vi "Teleop.vi"(10 "Match Info":T1={"Autonomous Elapsed Seconds"=0.0, "TeleOp Elapsed Seconds"=0.0, "Disabled Elapsed Seconds"=0.0, "Visited Autonomous"=FALSE, "Visited TeleOp"=FALSE, "Visited Disabled"=FALSE, "Autonomous Settings"={"Autonomous Style"=enum."Independent", "VI Refnum"=refnum}}, 11 "Call Context":T2) -> ()   [LabVIEW 2015]
doc: "This VI is called for each enabled TeleOp packet received from the DS. It is typically used to read from joysticks and other inputs and update I/O or setpoints for timed control loops. It should complete and return within 20 milliseconds or risk missing DS packets."
uses:
  <vilib>/Rock Robotics/WPI/DriverStation/WPI_DriverStationDerivedRobotMode.ctl
  <vilib>/Rock Robotics/WPI/DriverStation/WPI_DriverStationMatch Info.ctl
  <vilib>/Rock Robotics/WPI/Solenoid/WPI_SolenoidValue.ctl
  <vilib>/Rock Robotics/WPI/Utilities/WPI_GetSetVariantRefNum.vi
  <vilib>/Rock Robotics/Network Tables/NT Write Boolean Array.vi
  <vilib>/Rock Robotics/Network Tables/NT Write Numeric Array.vi
  <vilib>/Rock Robotics/WPI/RobotDrive/WPI_RobotDriveArcadeDrive_Standard(NoSaturation).vi
  <vilib>/Rock Robotics/WPI/Solenoid/Deprecated/WPI_SolenoidGetBool.vi
  <vilib>/Rock Robotics/WPI/Solenoid/WPI_SolenoidSetEnum.vi
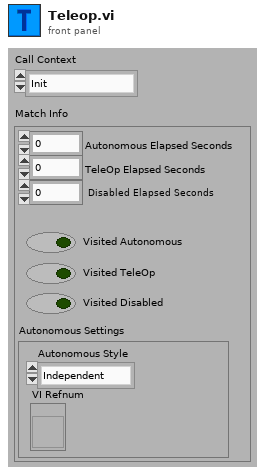
[diagram p1: front panel]
types:
  T1 = typedef "WPI_DriverStationMatch Info.ctl" = cluster{"Autonomous Elapsed Seconds":dbl, "TeleOp Elapsed Seconds":dbl, "Disabled Elapsed Seconds":dbl, "Visited Autonomous":bool, "Visited TeleOp":bool, "Visited Disabled":bool, "Autonomous Settings":cluster{"Autonomous Style":enum16{"Iterative", "Independent"}, "VI Refnum":refnum<vi>}}
  T2 = typedef "WPI_DriverStationDerivedRobotMode.ctl" = enum16{"Init", "Execute", "Stop"}
  T3 = typedef "WPI_SolenoidValue.ctl" = enum16{"Off", "On", "Forward", "Reverse"}
  T4 = typedef "WPI_RobotDriveDevRef.ctl" = cluster{"DevStatus":errorcluster, "Motors[]":T5[], "Square Inputs":bool, "Max Output":dbl}
  T5 = typedef "WPI_MotorControlDeviceRef.ctl" = cluster{"DeviceStatus":errorcluster, "Type":T6, "PWM":cluster{"PWM Channel":T7, "DeadBand":T8}, "CAN":cluster{"Device Number":u8, "Control Mode":T9, "Semaphore":T10, "Max Vout":dbl, "TalonSRX Control Mode":T11}, "Invert":bool}
  T6 = typedef "WPI_MotorControlType.ctl" = enum16{"PWM", "CAN", "CANTalonSRX"}
  T7 = typedef "FPGA_DIOPWMChannel.ctl" = enum8{"PWM 0", "PWM 1", "PWM 2", "PWM 3", "PWM 4", "PWM 5", "PWM 6", "PWM 7", "PWM 8", "PWM 9", "PWM MXP 0", "PWM MXP 1", "PWM MXP 2", "PWM MXP 3", "PWM MXP 4", "PWM MXP 5", "PWM MXP 6", "PWM MXP 7", "PWM MXP 8", "PWM MXP 9", "Invalid"}
  T8 = typedef "WPI_PWMDeadband.ctl" = cluster{"Name":string, "maxPositivePwm":i32, "minPositivePwm":i32, "centerPwm":i32, "maxNegativePwm":i32, "minNegativePwm":i32, "angularRange":u16}
  T9 = typedef "WPI_CANJaguar_ControlMode.ctl" = enum8{"Percent VBus", "Current", "Speed", "Position", "Voltage"}
  T10 = typedef "Semaphore RefNum" = refnum<k1>
  T11 = typedef "WPI_CANTalonSRX_APIControlMode.ctl" = enum8{"Percent VBus", "Speed", "Position", "Slave", "Unchanged / Invalid", "Voltage Compensation", "Current", "Motion Profile"}
  T12 = typedef "WPI_JoystickDevRef.ctl" = cluster{"Device":T13}
  T13 = typedef "WPI_JoystickDeviceEnum.ctl" = enum16{"USB 0", "USB 1", "USB 2", "USB 3", "USB 4", "USB 5"}
  T14 = cluster{"Buttons[0]":bool, "Buttons[1]":bool, "Buttons[2]":bool, "Buttons[3]":bool, "Buttons[4]":bool, "Buttons[5]":bool, "Buttons[6]":bool, "Buttons[7]":bool, "Buttons[8]":bool}
  T15 = cluster{"Axes[0]":dbl, "Axes[1]":dbl, "Axes[2]":dbl, "Axes[3]":dbl, "Axes[4]":dbl, "Axes[5]":dbl, "Axes[6]":dbl, "Axes[7]":dbl, "Axes[8]":dbl}
  T16 = typedef "WPI_SolenoidDevRef.ctl" = cluster{"DevStatus":errorcluster, "Pneumatics Control Module":u8, "Forward Solenoid Channel":T17, "Reverse Solenoid Channel":T17}
  T17 = typedef "WPI_SolenoidChannel.ctl" = enum8{"Solenoid 0", "Solenoid 1", "Solenoid 2", "Solenoid 3", "Solenoid 4", "Solenoid 5", "Solenoid 6", "Solenoid 7", "Invalid"}
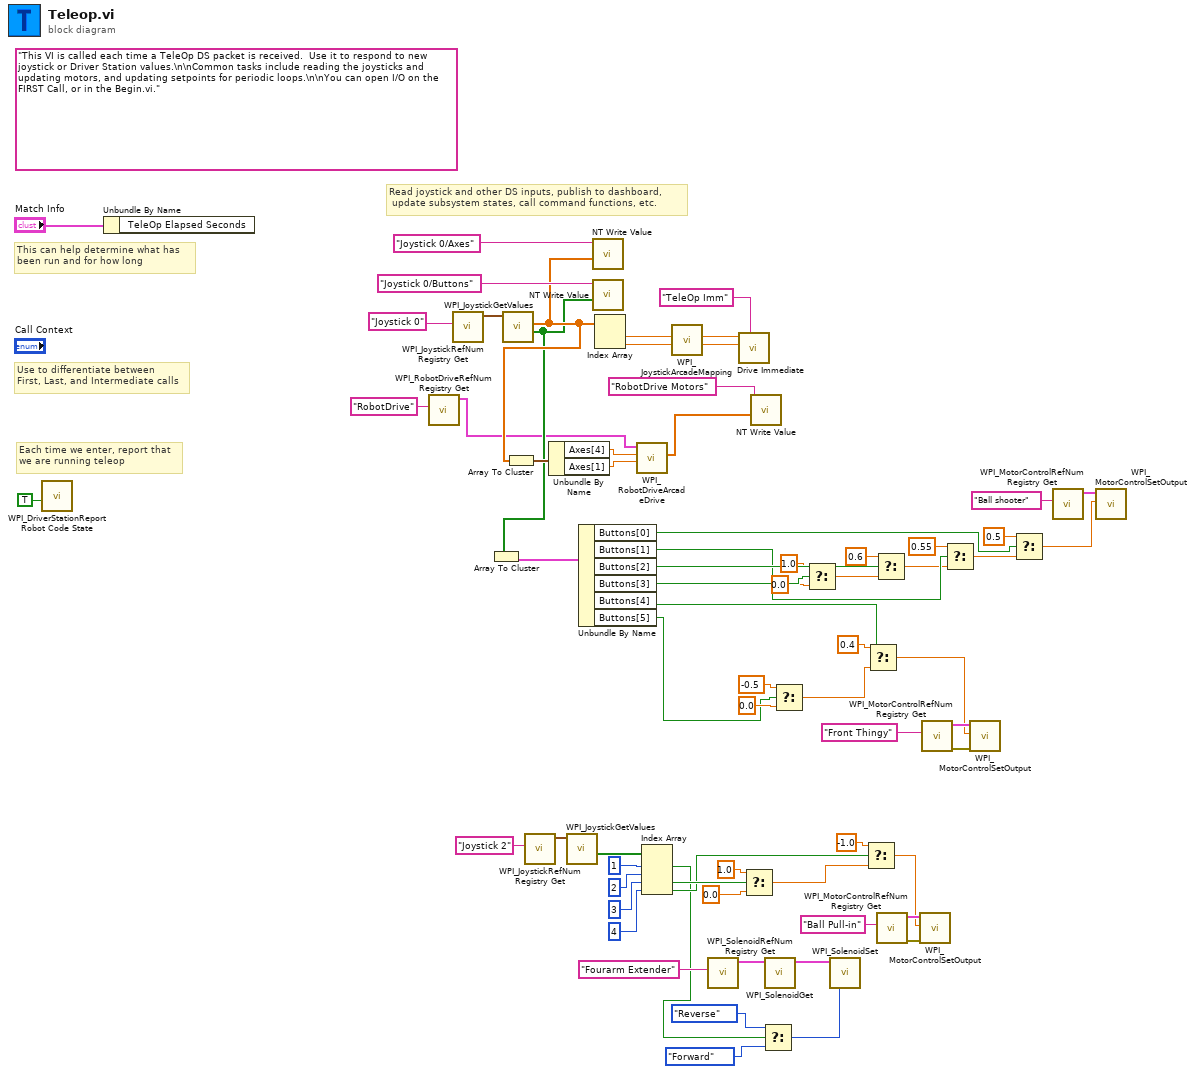
[diagram p0: block diagram]
diagram:
  (unwired) "This VI is called each time a TeleOp DS packet is received.  Use it to respond to new joystick or Driver Station values.\n\nCommon tasks include reading the joysticks and updating motors, and updating setpoints for periodic loops.\n\nYou can open I/O on the FIRST Call, or in the Begin.vi."
  # "Read joystick and other DS inputs, publish to dashboard,\n update subsystem states, call command functions, etc."
  # "Each time we enter, report that\nwe are running teleop"
  # "Use to differentiate between\nFirst, Last, and Intermediate calls"
  # "This can help determine what has\nbeen run and for how long"
  n1 = call <vilib>:"WPI_DriverStationReport Robot Code State.vi"("TeleOp"=TRUE ("Autonomous")) -> ()  [unwired: 10 in, 1 out]
  n2 = Unbundle By Name("Match Info") -> ()  [unwired: 1 out]
  n3 = call <vilib>:"WPI_RobotDriveRefNum Registry Get.vi"("refnum name"="RobotDrive" ("Name")) -> ("RobotDriveDevRef"=w31:T4)  [unwired: 9 in, 1 out]
  n4 = call <vilib>:"WPI_JoystickRefNum Registry Get.vi"("refnum name"="Joystick 0") -> ("JoystickDevRef"=w67:T12)  [unwired: 1 in, 9 out]
  n5 = call <vilib>:"WPI_JoystickGetValues.vi"("JoystickDevRef"=w67) -> ("Buttons"=w53:bool[], "Axes"=w59:dbl[])  [unwired: 6 in, 3 out]
  n6 = Array To Cluster(array=w53) -> (cluster=w52:T14)
  n7 = Array To Cluster(array=w59) -> (cluster=w58:T15)
  n8 = call <vilib>:"WPI_JoystickRefNum Registry Get.vi"("refnum name"="Joystick 2") -> ("JoystickDevRef"=w18:T12)  [unwired: 9 in, 1 out]
  n9 = Unbundle By Name(w58) -> ("Axes[4]"=w57:dbl, "Axes[1]"=w56:dbl)
  n10 = call <vilib>:"WPI_JoystickGetValues.vi"("JoystickDevRef"=w18) -> ("Buttons"=w25:bool[])  [unwired: 6 in, 4 out]
  n11 = Unbundle By Name(w52) -> ("Buttons[0]"=w45:bool, "Buttons[1]"=w47:bool, "Buttons[2]"=w48:bool, "Buttons[3]"=w50:bool, "Buttons[4]"=w34:bool, "Buttons[5]"=w28:bool)
  n12 = call-poly <vilib>:"NT Write Value.vi"("Numeric Array"=w59, "Name"="Joystick 0/Axes") -> ()  [unwired: 9 in, 1 out]
  n13 = call-poly <vilib>:"NT Write Value.vi"("Boolean Array"=w53, "Name"="Joystick 0/Buttons") -> ()  [unwired: 9 in, 1 out]
  n14 = Index Array(array=w59) -> (element #1=w63:dbl, element #2=w62:dbl)  [unwired: 2 in]
  n15 = call-poly <vilib>:"WPI_RobotDriveArcadeDrive.vi"("Y axis value"=w56, "X axis value"=w57, "RobotDriveDevRef"=w31) -> ("Motor Values"=w55:dbl[])  [unwired: 6 in, 2 out]
  n16 = Index Array(array=w25, index #1=1 ("index"), index #2=2 ("index"), index #3=3 ("index"), index #4=4 ("index")) -> (element #1=w3:bool, element #3=w10:bool, element #4=w6:bool)  [unwired: 1 out]
  n17 = call <vilib>:"WPI_JoystickArcadeMapping.vi"("Y axis value"=w62, "X axis value"=w63) -> ("Right Motor Value"=w64:dbl, "Left Motor Value"=w65:dbl)  [unwired: 8 in]
  n18 = call <vilib>:"WPI_SolenoidRefNum Registry Get.vi"("refnum name"="Fourarm Extender") -> ("SolenoidDevRef"=w22:T16)  [unwired: 9 in, 1 out]
  n19 = call "Drive Immediate.vi"("Description"="TeleOp Imm", "Right Setpoint"=w64, "Left Setpoint"=w65) -> ()  [unwired: 8 in, 1 out]
  n20 = Select(t=1.0, s=w10, f=0.0) -> (s? t:f=w7:dbl)
  n21 = call-poly <vilib>:"NT Write Value.vi"("Numeric Array"=w55, "Name"="RobotDrive Motors") -> ()  [unwired: 9 in, 1 out]
  n22 = Select(t=WPI_SolenoidValue."Reverse" ("Value"), s=w3, f=WPI_SolenoidValue."Forward" ("Value")) -> (s? t:f=w4:T3)
  n23 = call-poly <vilib>:"WPI_SolenoidGet.vi"("SolenoidDevRef"=w22) -> ("SolenoidDevRef"=w20:T16)  [unwired: 8 in, 2 out]
  n24 = Select(t=-0.5, s=w28, f=0.0) -> (s? t:f=w27:dbl)
  n25 = Select(t=1.0, s=w50, f=0.0) -> (s? t:f=w49:dbl)
  n26 = call-poly <vilib>:"WPI_SolenoidSet.vi"("Value"=w4, "SolenoidDevRef"=w20) -> ()  [unwired: 8 in, 2 out]
  n27 = Select(t=-1.0, s=w6, f=w7) -> (s? t:f=w5:dbl)
  n28 = Select(t=0.4, s=w34, f=w27) -> (s? t:f=w26:dbl)
  n29 = Select(t=0.6, s=w48, f=w49) -> (s? t:f=w46:dbl)
  n30 = call <vilib>:"WPI_MotorControlRefNum Registry Get.vi"("refnum name"="Ball Pull-in") -> ("error out"=w13:errorcluster, "MotorControlDevRef"=w14:T5)  [unwired: 9 in]
  n31 = call <vilib>:"WPI_MotorControlSetOutput.vi"("error in (no error)"=w13, "Output"=w5, "MotorControlDevRef"=w14) -> ()  [unwired: 6 in, 3 out]
  n32 = call <vilib>:"WPI_MotorControlRefNum Registry Get.vi"("refnum name"="Front Thingy") -> ("error out"=w37:errorcluster, "MotorControlDevRef"=w36:T5)  [unwired: 9 in]
  n33 = Select(t=0.55, s=w47, f=w46) -> (s? t:f=w44:dbl)
  n34 = call <vilib>:"WPI_MotorControlSetOutput.vi"("error in (no error)"=w37, "Output"=w26, "MotorControlDevRef"=w36) -> ()  [unwired: 6 in, 3 out]
  n35 = Select(t=0.5, s=w45, f=w44) -> (s? t:f=w1:dbl)
  n36 = call <vilib>:"WPI_MotorControlRefNum Registry Get.vi"("refnum name"="Ball shooter") -> ("MotorControlDevRef"=w51:T5)  [unwired: 9 in, 1 out]
  n37 = call <vilib>:"WPI_MotorControlSetOutput.vi"("Output"=w1, "MotorControlDevRef"=w51) -> ()  [unwired: 7 in, 3 out]
